vi "认识移位寄存器.vi"() -> ()   [LabVIEW 2018]
panel:
  out "?":u8(slide) scale=0.0..11.0
  out "数值 3":dbl
  out "数值 2":dbl
  out "数值":dbl
  out "字符串":string="移位寄存器"
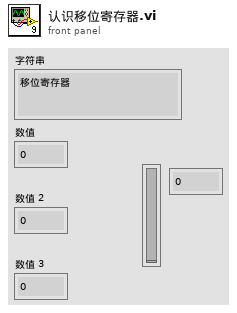
[diagram p1: front panel]
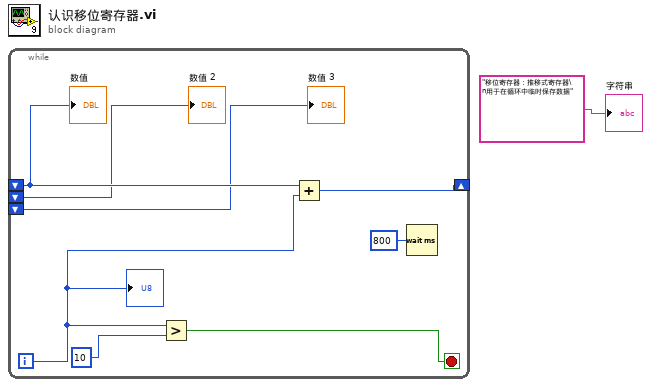
[diagram p0: block diagram]
diagram:
  n1 = while {
    shift-right: [w7] -> _
    shift-left: _ -> [w6]
    shift-left: _ -> [w5]
    shift-left: _ -> [w4]
    i -> [w2]
    stop <- w8 stop-if-true
    n2 = Greater?(x=w2, y=10) -> (0:w8:bool)
    n3 = Add(x=w6, y=w2) -> (x+y=w7:i32)
    n4 = Wait (ms)(milliseconds to wait=u32 800 ("等待时间（毫秒）")) -> ()  [unwired: 1 out]
    "数值" <- w6
    "数值 2" <- w5
    "数值 3" <- w4
    "?" <- w2
  }
  "字符串" <- "移位寄存器：推移式寄存器\n用于在循环中临时保存数据"
